vi "Verify Chan Res Cal Test V2.vi"(7 "Device Name":string, 8 "error in":errorcluster, 9 "Resistance":T1, 10 "nDelayValue":i32, 11 "nScale":i32) -> (0 "error out":errorcluster, 3 "Channel Ohms Result":dbl)   [LabVIEW 2013]
uses:
  DAQ/Resistances.ctl
  DAQ/Relay Modes.ctl
  DAQ/Channels_v2.ctl
panel:
  in  "Delay Time (s)":dbl=1.0
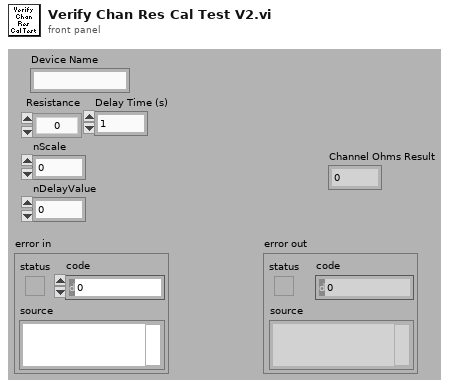
[diagram p1: front panel]
types:
  T1 = typedef "Resistances.ctl" = enum16{"0", "20", "40", "200", "400", "2k", "4K", "20k", "40K", "200k", "400K", "2M", "4M"}
  T2 = typedef "Channels_v2.ctl" = enum16{"All Off", "Channel 4", "Channel 3", "4,3", "Channel 2", "4,2", "3,2", "4,3,2,", "Channel 1", "4,1", "3,1", "4,3,1", "2,1", "4,2,1", "3,2,1", "All On"}
  T3 = typedef "Relay Modes.ctl" = enum16{"All Off", "Short", "Ohms", "Fluke", "Daq AO 0"}
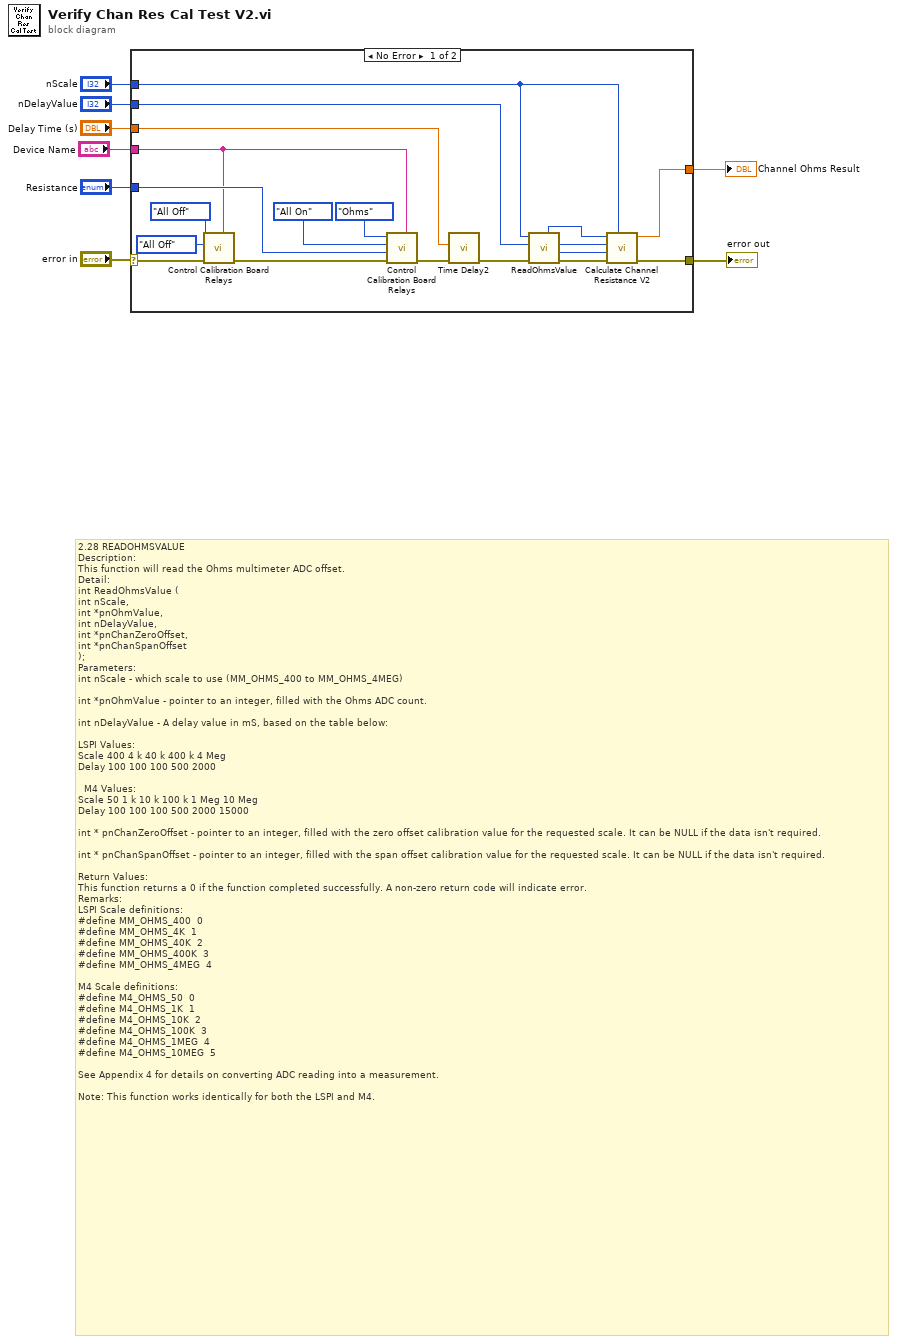
[diagram p0: block diagram]
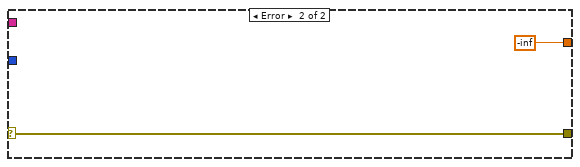
[diagram p2: hidden frame]
diagram:
  # "2.28\tREADOHMSVALUE\nDescription:\nThis function will read the Ohms multimeter ADC offset.\nDetail:\nint ReadOhmsValue (\nint nScale, \nint *pnOhmValue, \nint nDelayValue, \nint *pnChanZeroOffset,\nint *pnChanSpanOffset\n);\nParameters:\nint nScale - which scale to use (MM_OHMS_400 to MM_OHMS_4MEG)\n\nint *pnOhmValue - pointer to an integer, filled with the Ohms ADC count.\n\nint nDelayValue - A delay value in mS, based on the table below:\n\nLSPI Values:\nScale\t400\t4 k\t40 k\t400 k\t4 Meg\nDelay\t100\t100\t100\t500\t2000\n\n\t\tM4 Values:\nScale\t50\t1 k\t10 k\t100 k\t1 Meg\t10 Meg\nDelay\t100\t100\t100\t500\t2000\t15000\n\nint * pnChanZeroOffset - pointer to an integer, filled with the zero offset calibration value for the requested scale. It can be NULL if the data isn't required.\n\nint * pnChanSpanOffset - pointer to an integer, filled with the span offset calibration value for the requested scale. It can be NULL if the data isn't required.\n\nReturn Values:\nThis function returns a 0 if the function completed successfully. A non-zero return code will indicate error. \nRemarks:\nLSPI Scale definitions:\n#define MM_OHMS_400\t\t0\n#define MM_OHMS_4K\t\t1\n#define MM_OHMS_40K\t\t2\n#define MM_OHMS_400K\t\t3\n#define MM_OHMS_4MEG\t\t4\n\nM4 Scale definitions:\n#define M4_OHMS_50\t\t0\n#define M4_OHMS_1K\t\t1\n#define M4_OHMS_10K\t\t2\n#define M4_OHMS_100K\t\t3\n#define M4_OHMS_1MEG\t\t4\n#define M4_OHMS_10MEG\t\t5\n\nSee Appendix 4 for details on converting ADC reading into a measurement.\n\nNote: This function works identically for both the LSPI and M4."
  n1 = case shown="No Error" "error in" {
    selector: "error in" -> [w13 w29]
    tunnel: [w23 w29] -> w7
    tunnel: [w22 -inf] -> w6
    tunnel: "nDelayValue" -> [w21 _]
    tunnel: "nScale" -> [w20 _]
    tunnel: "Resistance" -> [w18 _]
    tunnel: "Delay Time (s)" -> [w15 _]
    tunnel: "Device Name" -> [w11 _]
    frame No Error {
      n2 = call "Control Calibration Board Relays.vi"("Device Name"=w11, "error in"=w13, "Channels"=Channels_v2."All Off", "Mode"=Relay_Modes."All Off") -> ("error out"=w12:errorcluster)  [unwired: 7 in]
      n3 = call "Control Calibration Board Relays.vi"("Device Name"=w11, "error in"=w12, "Resistance"=w18, "Channels"=Channels_v2."All On", "Mode"=Relay_Modes."Ohms") -> ("error out"=w17:errorcluster)  [unwired: 6 in]
      n4 = call "Time Delay2"("error in (no error)"=w17, "Delay Time (s)"=w15) -> ("error out"=w16:errorcluster)  [unwired: 9 in]
      n5 = call "ReadOhmsValue.vi"("error in"=w16, "nDelayValue"=w21, "nScale"=w20) -> ("error out"=w24:errorcluster, "*pnChanSpanOffset"=w25:i32, "*pnChanZeroOffset"=w26:i32, "*pnOhmValue"=w27:i32)  [unwired: 4 in, 1 out]
      n6 = call "Calculate Channel Resistance V2.vi"("Scale"=w20, "error in (no error)"=w24, "ChanSpanOffset"=w25, "ChanZeroOffset"=w26, "ChanValue"=w27) -> ("error out"=w23:errorcluster, "Channel Ohms Result"=w22:dbl)  [unwired: 5 in]
    }
    frame Error {
    }
  }
  "error out" <- w7
  "Channel Ohms Result" <- w6
